vi "process selected file.vi"(8 "error in":errorcluster, 11 "Cluster in":T1={"This VI Ref"=refnum, "Test VI"=refnum, "Q Ref"=refnum, "UE"=refnum, "Data"=variant, "Timeout"=-1, "Path List[]"=[], "Status"="", "Counter"=0, "Config"={"Source Path"=path "", "Dest Path"=path "", "Log Path"=path "", "Move?"=FALSE, "Log?"=FALSE, "Scanners"=[], "Excude Folders"=[], "Jpg?"=FALSE, "Default path"=path "", "Extended?"=FALSE, "Mode"=enum."Move"}, "Total"=0, "Config Path"=path "", "exif info"={"Make"="Canon\u0000", "Model"="Canon PowerShot A495\u0000", "Orientation"=0, "Date"=timestamp(0 s since 1904-01-01), "Width"=0, "Height"=0, "Square?"=FALSE, "File Name"="Canon\u0000", "Extension"="Canon\u0000", "Valid?"=FALSE, "Path"=path "", "size"=0, "No Ext?"=FALSE, "prefix?"=FALSE, "String"="", "Name Type"=enum."Event Sufix"}, "app operation"=enum."Start", "Log Ref"=refnum, "Start Time"=0.0, "Pause Time"=0.0, "Argument?"=FALSE, "Argument path"=path "", "Identical"=FALSE, "File.lvclass"=refnum}) -> (0 "error out":errorcluster, 3 "Cluster out":T1={"This VI Ref"=refnum, "Test VI"=refnum, "Q Ref"=refnum, "UE"=refnum, "Data"=variant, "Timeout"=-1, "Path List[]"=[], "Status"="", "Counter"=0, "Config"={"Source Path"=path "", "Dest Path"=path "", "Log Path"=path "", "Move?"=FALSE, "Log?"=FALSE, "Scanners"=[], "Excude Folders"=[], "Jpg?"=FALSE, "Default path"=path "", "Extended?"=FALSE, "Mode"=enum."Move"}, "Total"=0, "Config Path"=path "", "exif info"={"Make"="Canon\u0000", "Model"="Canon PowerShot A495\u0000", "Orientation"=0, "Date"=timestamp(0 s since 1904-01-01), "Width"=0, "Height"=0, "Square?"=FALSE, "File Name"="Canon\u0000", "Extension"="Canon\u0000", "Valid?"=FALSE, "Path"=path "", "size"=0, "No Ext?"=FALSE, "prefix?"=FALSE, "String"="", "Name Type"=enum."Event Sufix"}, "app operation"=enum."Start", "Log Ref"=refnum, "Start Time"=0.0, "Pause Time"=0.0, "Argument?"=FALSE, "Argument path"=path "", "Identical"=FALSE, "File.lvclass"=refnum})   [LabVIEW 2023, in "User Interface.lvlib"]
uses:
  User Interface.lvlib
  Controls/main consumer cluster.ctl
  File Classes/File/File.lvclass
  Controls/configuration cluster.ctl
  File Classes/Controls/exif data cluster.ctl
  File Classes/Controls/rename type enum.ctl
  Controls/app operation state enum.ctl
  File Classes/File Classes.lvlib
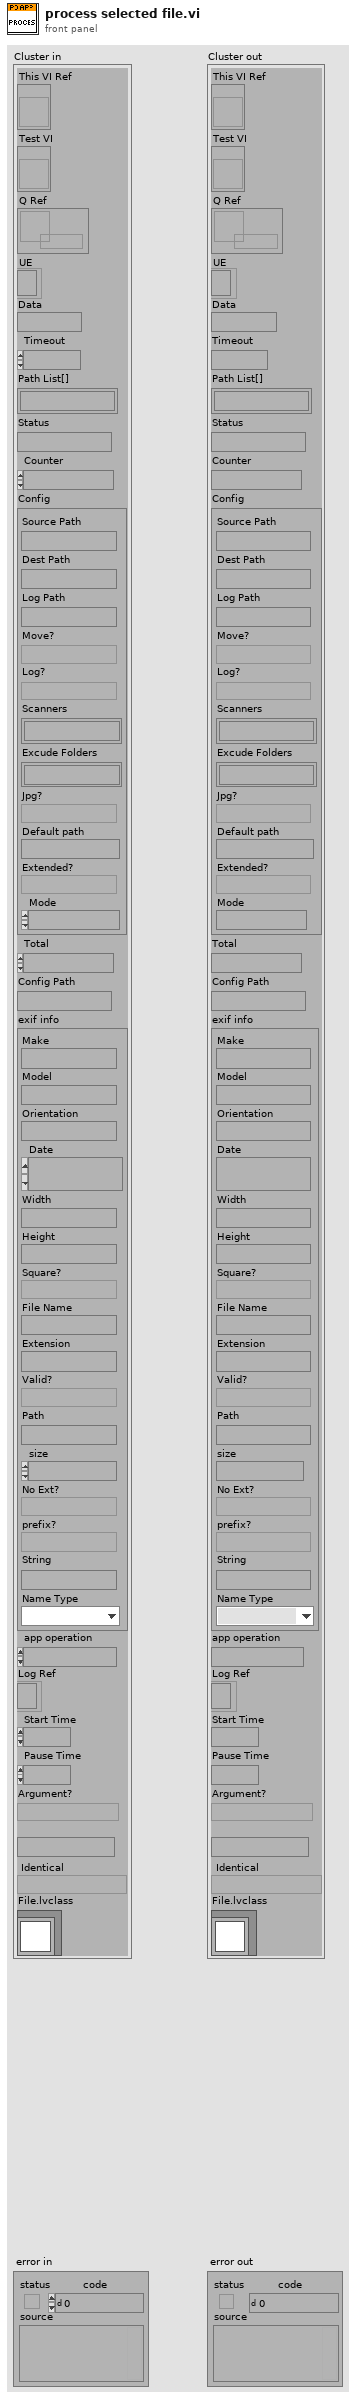
[diagram p1: front panel]
types:
  T1 = typedef "User Interface.lvlib/main consumer cluster.ctl" = cluster{"This VI Ref":refnum<vi>, "Test VI":refnum<vi>, "Q Ref":refnum<queue>, "UE":refnum<event-registration>, "Data":variant, "Timeout":i32, "Path List[]":path[], "Status":string, "Counter":i32, "Config":T2, "Total":i32, "Config Path":path, "exif info":T3, "app operation":T5, "Log Ref":refnum<file>, "Start Time":dbl, "Pause Time":dbl, "Argument?":bool, "Argument path":path, "Identical":bool, "File.lvclass":refnum<class "File.lvclass">}
  T2 = typedef "User Interface.lvlib/configuration cluster.ctl" = cluster{"Source Path":path, "Dest Path":path, "Log Path":path, "Move?":bool, "Log?":bool, "Scanners":string[], "Excude Folders":string[], "Jpg?":bool, "Default path":path, "Extended?":bool, "Mode":enum16{"Copy (Default)", "Move", "Rename"}}
  T3 = typedef "File Classes.lvlib/exif data cluster.ctl" = cluster{"Make":string, "Model":string, "Orientation":u16, "Date":timestamp, "Width":u16, "Height":u16, "Square?":bool, "File Name":string, "Extension":string, "Valid?":bool, "Path":path, "size":i64, "No Ext?":bool, "prefix?":bool, "String":string, "Name Type":T4}
  T4 = typedef "File Classes.lvlib/rename type enum.ctl" = enum16{"Date & Time (Default)", "Model Sufix", "Event Sufix", "Model & Event Sufix"}
  T5 = typedef "User Interface.lvlib/app operation state enum.ctl" = enum16{"Start", "Stop", "Pause", "Resume"}
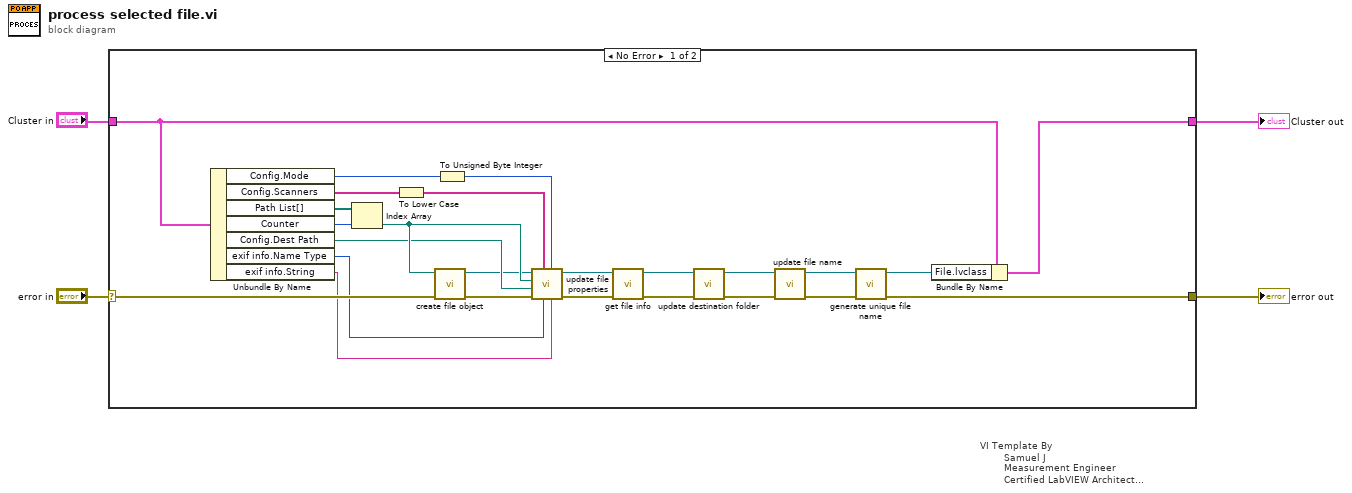
[diagram p0: block diagram]
diagram:
  n1 = case "VI Template By\n        Samuel J\n        Measurement Engineer\n        Certified LabVIEW Architect\n        Vestas Technology R&D Chennai" shown="No Error" "error in" {
    selector: "error in" -> [w28 w31]
    tunnel: [w15 w31] -> w3
    tunnel: [w29 w30] -> w2
    tunnel: "Cluster in" -> [w26 w30]
    frame No Error {
      n2 = Unbundle By Name(w26) -> ("Config.Mode"=w8:enum16{"Copy (Default)", "Move", "Rename"}, "Config.Scanners"=w23:string[], "Path List[]"=w25:path[], "Counter"=w27:i32, "Config.Dest Path"=w22:path, "exif info.Name Type"=w6:T4, "exif info.String"=w5:string)
      n3 = Index Array(array=w25, index=w27) -> (element=w24:path)
      n4 = To Lower Case(string=w23) -> (all lower case string=w13:string[])
      n5 = call "create file object.vi"("error in (no error)"=w28, "file path"=w24) -> ("error out"=w20:errorcluster, "reference out"=w21:refnum<class "File.lvclass">)  [unwired: 8 in]
      n6 = To Unsigned Byte Integer(number=w8) -> (unsigned 8bit integer=w7:u8)
      n7 = call "update file properties.vi"("event name"=w5, "mode"=w7, "file format"=w6, "scanner[]"=w13, "error in (no error)"=w20, "destination path"=w22, "file path"=w24, "File in"=w21) -> ("error out"=w18:errorcluster, "File out"=w19:refnum<class "File.lvclass">)  [unwired: 2 in]
      n8 = call-dynamic "get file info.vi"("error in (no error)"=w18, "File in"=w19) -> ("error out"=w16:errorcluster, "File out"=w17:refnum<class "File.lvclass">)  [unwired: 8 in]
      n9 = call-dynamic "update destination folder.vi"("error in (no error)"=w16, "File in"=w17) -> ("error out"=w11:errorcluster, "File out"=w12:refnum<class "File.lvclass">)  [unwired: 8 in]
      n10 = call-dynamic "update file name.vi"("error in (no error)"=w11, "File in"=w12) -> ("error out"=w9:errorcluster, "File out"=w10:refnum<class "File.lvclass">)  [unwired: 8 in]
      n11 = call-dynamic "generate unique file name.vi"("error in (no error)"=w9, "File in"=w10) -> ("error out"=w15:errorcluster, "File out"=w14:refnum<class "File.lvclass">)  [unwired: 8 in]
      n12 = Bundle By Name(cluster=w26, "File.lvclass"=w14) -> (w29:T1)
    }
    frame Error {
    }
  }
  "error out" <- w3
  "Cluster out" <- w2
